vi "Get Python.vi"(8 "error in (no error)":errorcluster, 11 "PyServer in":refnum<class "PyServer.lvclass">) -> (0 "error out":errorcluster, 2 "resulting string":string, 3 "PyServer out":refnum<class "PyServer.lvclass">)   [LabVIEW 2025, in "Tools.lvlib" / "PyServer.lvclass"]
uses:
  PyServer.lvclass
  PyServer.lvclass/PyServer.ctl
  PyTool/PyTool.lvclass
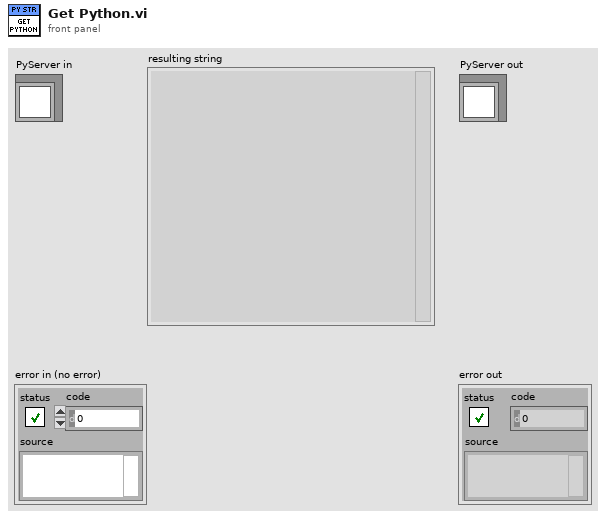
[diagram p1: front panel]
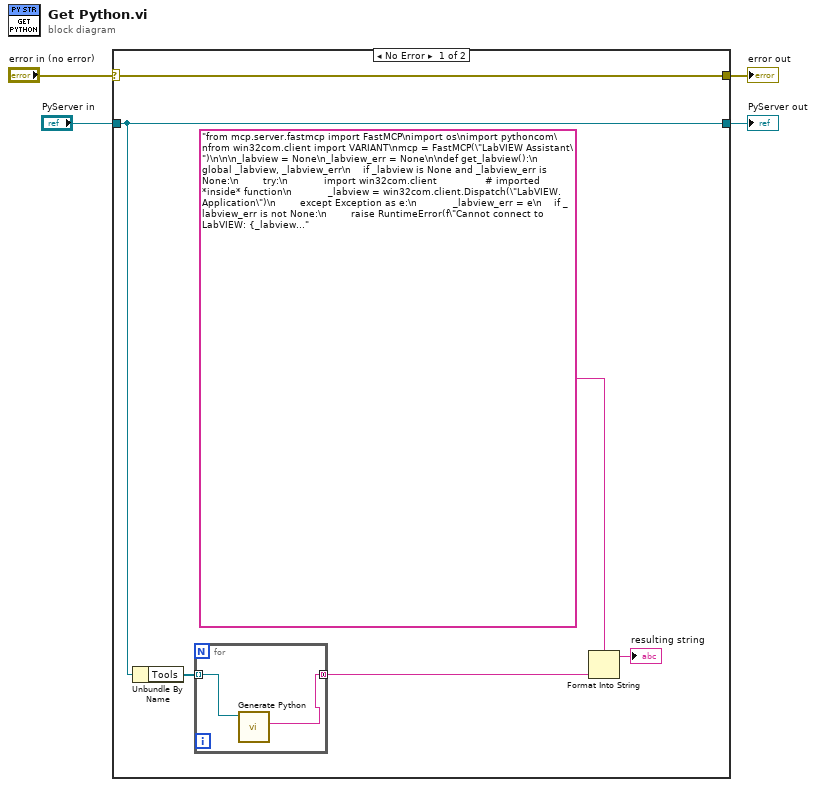
[diagram p0: block diagram]
diagram:
  n1 = case shown="No Error" "error in (no error)" {
    selector: "error in (no error)" -> [w10 w14]
    tunnel: [w10 w14] -> w3
    tunnel: [w9 w13] -> w1
    tunnel: "PyServer in" -> [w9 w13]
    frame No Error {
      n2 = Unbundle By Name(w9) -> ("Tools"=w7:refnum<class "PyTool.lvclass">[])
      n3 = for {
        tunnel: w7 -> [w12] mode=indexing
        tunnel: [w11] -> w6 mode=concatenating
        n4 = call "Generate Python.vi"("PyTool in"=w12) -> ("Python Code"=w11:string)  [unwired: 8 in, 2 out]
      }
      n5 = Format Into String(format string="from mcp.server.fastmcp import FastMCP\nimport os\nimport pythoncom\nfrom win32com.client import VARIANT\nmcp = FastMCP(\"LabVIEW Assistant\")\n\n\n_labview = None\n_labview_err = None\n\ndef get_labview():\n    global _labview, _labview_err\n    if _labview is None and _labview_err is None:\n        try:\n            import win32com.client                # imported *inside* function\n            _labview = win32com.client.Dispatch(\"LabVIEW.Application\")\n        except Exception as e:\n            _labview_err = e\n    if _labview_err is not None:\n        raise RuntimeError(f\"Cannot connect to LabVIEW: {_labview_err}\")\n    return _labview\n\n\n@mcp.tool()\ndef echo(text: str) -> str:\n    \"\"\"Echoes back the provided text.\"\"\"\n    return f\"You said: {text}\"\n\n%s\n\nif __name__ == \"__main__\":\n    mcp.run()\n", w6) -> (resulting string=→"resulting string":string)  [unwired: 2 in, 1 out]
    }
    frame Error {
    }
  }
  "error out" <- w3
  "PyServer out" <- w1
